vi "SubVI RX Make Toeplitz.vi"(6 "column":cdb[](array[numeric]), 7 "row":cdb[](array[numeric])) -> (3 "Toeplitz Array":cdb[][](array[numeric]))   [LabVIEW 2015]
panel:
  # "Generate a Toeplitz array from initial row and column"
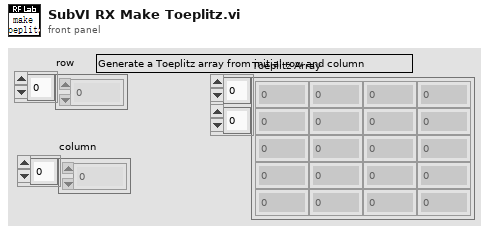
[diagram p1: front panel]
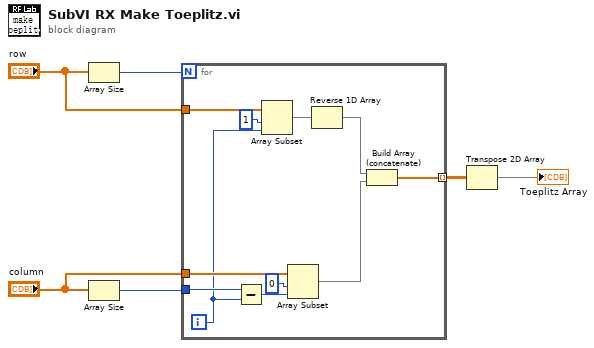
[diagram p0: block diagram]
diagram:
  n1 = Array Size(array="row") -> (size(s)=w6:i32)
  n2 = Array Size(array="column") -> (size(s)=w3:i32)
  n3 = for {
    N: w6 -> [_]
    tunnel: "row" -> [w11]
    tunnel: "column" -> [w15]
    tunnel: w3 -> [w17]
    tunnel: [w7] -> w2 mode=indexing
    i -> [w13]
    n4 = Subtract(x=w17, y=w13) -> (x-y=w16:i32)
    n5 = Array Subset(array=w11, index=1, length=w13) -> (w10:cdb[])
    n6 = Array Subset(array=w15, index=0, length=w16) -> (w8:cdb[])
    n7 = Reverse 1D Array(array=w10) -> (reversed array=w9:cdb[])
    n8 = Build Array (concatenate)(w9, w8) -> (w7:cdb[])
  }
  n9 = Transpose 2D Array(2D array=w2) -> (transposed array=→"Toeplitz Array":cdb[][])
